vi "Example.vi"() -> ()   [LabVIEW 2019]
uses:
  Scope Driver/Typedef/Horizontal Settings.ctl
  Scope Driver/Typedef/TimeSetting.ctl
  Scope Driver/Typedef/Metadata/[Meta]SetupInfoTrigger.ctl
  Scope Driver/Typedef/Vertical Settings.ctl
  Scope Driver/Typedef/Channel Selection.ctl
  Scope Driver/Typedef/Coupling.ctl
  Scope Driver/Typedef/RangeSetting.ctl
  Scope Driver/Typedef/Metadata/[Meta]SetupInfoV.ctl
  Scope Driver/Typedef/TriggerData.ctl
  Scope Driver/Typedef/Edge.ctl
  Scope Driver/Typedef/Metadata/[Meta]SetupInfoH.ctl
  SmartScopeDriver.lvclass
  Scope Driver/LabNation Scope Driver.lvlib
panel:
  out "[Meta]SetupInfoH":T1
  out "Waveform Graph":dbl[](array[numeric])
  out "created new?":bool
  in  "error in (no error)":errorcluster
  in  "Session  Name ()":string
  in  "Trigger Config":T2={"Channel"=enum."chn B", "Edge"=0, "Level[V]"=0.5} {"Edge" items=["RISING", "FALLING", "ANY"]}
  out "[Meta]SetupInfoV":T5
  in  "Vertical Settings":T6={"ChannelSelection"=enum."chn A", "Coupling"=0, "Offset[V]"=0.0, "V/div"=4.0} {"V/div" scale=0.0..6.0; "Coupling" items=["AC", "DC"]}
  out "[Meta]SetupInfoTrigger":T9
  in  "Horizontal Settings":T10={"Time/div"=0.01, "Trigger Holdoff"=0.0} {"Time/div" scale=0.0001..1.0 scale format="%#_8g"}
  out "error out":errorcluster
  in  "force destroy? (F)":bool
  in  "stop":bool
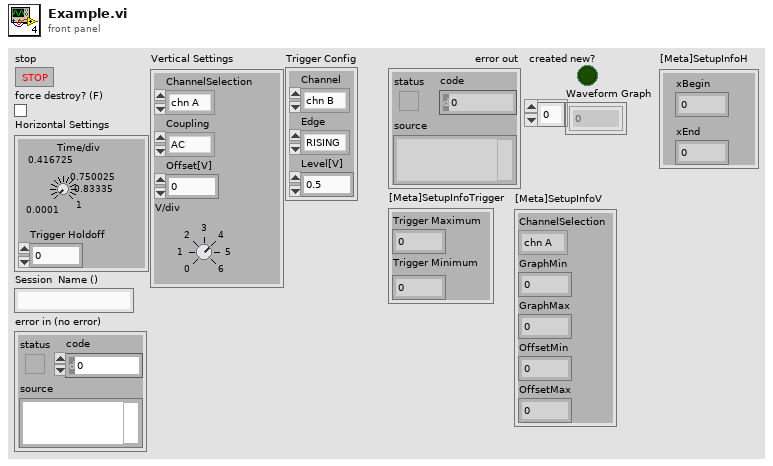
[diagram p1: front panel]
types:
  T1 = typedef "LabNation Scope Driver.lvlib/[Meta]SetupInfoH.ctl" = cluster{"xBegin":dbl, "xEnd":dbl}
  T2 = typedef "LabNation Scope Driver.lvlib/TriggerData.ctl" = cluster{"Channel":T3, "Edge":T4, "Level[V]":sgl}
  T3 = typedef "LabNation Scope Driver.lvlib/Channel Selection.ctl" = enum16{"chn A", "chn B"}
  T4 = typedef "LabNation Scope Driver.lvlib/Edge.ctl" = i32
  T5 = typedef "LabNation Scope Driver.lvlib/[Meta]SetupInfoV.ctl" = cluster{"ChannelSelection":T3, "GraphMin":dbl, "GraphMax":dbl, "OffsetMin":dbl, "OffsetMax":dbl}
  T6 = typedef "LabNation Scope Driver.lvlib/Vertical Settings.ctl" = cluster{"ChannelSelection":T3, "Coupling":T7, "Offset[V]":dbl, "V/div":T8}
  T7 = typedef "LabNation Scope Driver.lvlib/Coupling.ctl" = i32
  T8 = typedef "LabNation Scope Driver.lvlib/RangeSetting.ctl" = dbl
  T9 = typedef "LabNation Scope Driver.lvlib/[Meta]SetupInfoTrigger.ctl" = cluster{"Trigger Maximum":dbl, "Trigger Minimum":dbl}
  T10 = typedef "LabNation Scope Driver.lvlib/Horizontal Settings.ctl" = cluster{"Time/div":T11, "Trigger Holdoff":dbl}
  T11 = typedef "LabNation Scope Driver.lvlib/TimeSetting.ctl" = dbl
  T12 = typedef "SmartScopeDriver.lvclass/Session Handle.ctl" = refnum<data-value>
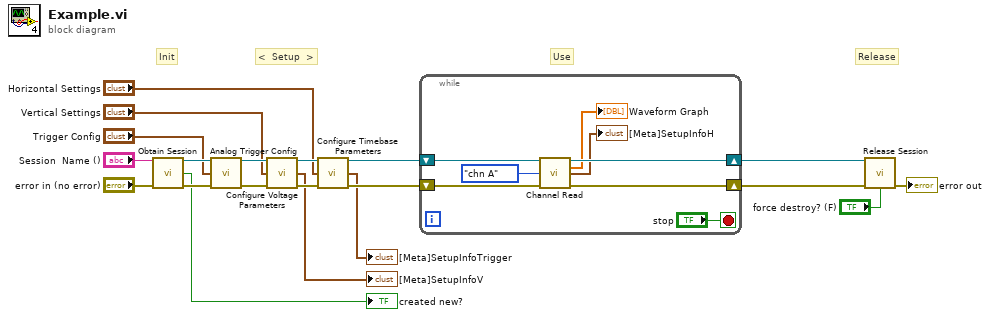
[diagram p0: block diagram]
diagram:
  # "Release"
  # "Use"
  # "<  Setup  >"
  # "Init"
  n1 = call "Obtain Session.vi"("Session  Name ()"="Session  Name ()", "error in (no error)"="error in (no error)") -> ("Session Handle"=w15:T12, "created new?"=→"created new?":bool, "error out"=w14:errorcluster)  [unwired: 11 in]
  n2 = call "Analog Trigger Config.vi"("Session Handle in"=w15, "Trigger Config"="Trigger Config", "error in (no error)"=w14) -> ("Session Handle out"=w16:T12, "error out"=w13:errorcluster)  [unwired: 11 in]
  n3 = call "Configure Voltage Parameters.vi"("Session Handle in"=w16, "Vertical Settings"="Vertical Settings", "error in (no error)"=w13) -> ("Session Handle out"=w17:T12, "[Meta]SetupInfoV"=→"[Meta]SetupInfoV":T5, "error out"=w12:errorcluster)  [unwired: 10 in]
  n4 = call "Configure Timebase Parameters.vi"("Session Handle in"=w17, "Horizontal Settings"="Horizontal Settings", "error in (no error)"=w12) -> ("Session Handle out"=w18:T12, "[Meta]SetupInfoTrigger"=→"[Meta]SetupInfoTrigger":T9, "error out"=w11:errorcluster)  [unwired: 10 in]
  n5 = while {
    shift-right: [w28] -> w20
    shift-left: w18 -> [w26]
    shift-right: [w27] -> w19
    shift-left: w11 -> [w25]
    stop <- "stop" stop-if-true
    n6 = call "Channel Read.vi"("Session Handle in"=w26, "ChannelSelection"=Channel_Selection."chn A", "error in (no error)"=w25) -> ("Session Handle out"=w28:T12, "Waveform Graph"=→"Waveform Graph":dbl[], "[Meta]SetupInfoH"=→"[Meta]SetupInfoH":T1, "error out"=w27:errorcluster)  [unwired: 9 in]
  }
  n7 = call "Release Session.vi"("Session Handle"=w20, "error in (no error)"=w19, "force destroy? (F)"="force destroy? (F)") -> ("error out"=→"error out":errorcluster)  [unwired: 12 in]
